vi "Time Above Threshold.vi"(3 "Current Value":dbl, 5 "Threshold":dbl) -> (1 "Time Above":u32)   [LabVIEW 2018]
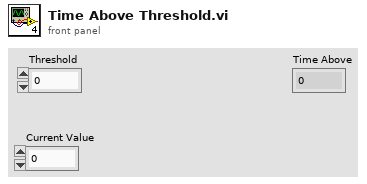
[diagram p1: front panel]
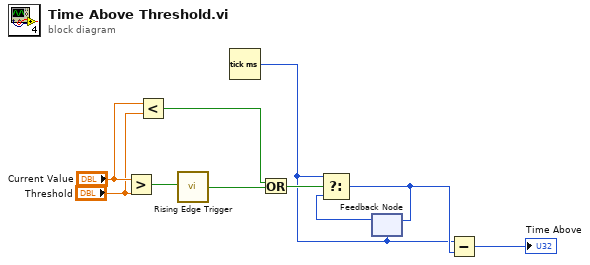
[diagram p0: block diagram]
diagram:
  n1 = Greater?(x="Current Value", y="Threshold") -> (0:w8:bool)
  n2 = Less?(x="Current Value", y="Threshold") -> (x < y?=w6:bool)
  n3 = call "Rising Edge Trigger.vi"("Raw Signal"=w8) -> ("Trigger"=w7:bool)
  n4 = Tick Count (ms)() -> (millisecond timer value=w2:u32)
  n5 = Or(x=w6, y=w7) -> (x .or. y?=w5:bool)
  n6 = feedback #1(w2) -> (w4:u32)
  n7 = Select(t=w2, s=w5, f=w4) -> (s? t:f=w3:u32)
  n8 = feedback-in #1(w3) -> ()
  n9 = Subtract(x=w2, y=w3) -> (x-y=→"Time Above":u32)
